vi "kill broken bundle.vi"(8 "error in":errorcluster, 11 "VI in":refnum<vi>) -> (0 "error out":errorcluster)   [LabVIEW 2013, in "FixedChannelTBModuleDecideFeatures.lvclass"]
uses:
  FixedChannelTBModuleDecideFeatures.lvclass
  <vilib>/Utility/traverseref.llb/TRef TravTarget.ctl
  <vilib>/Utility/traverseref.llb/VI Scripting - Traverse.lvlib
  <vilib>/Utility/VariantDataType/VariantType.lvlib
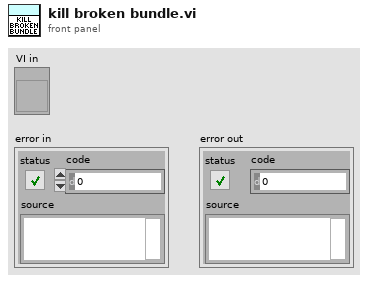
[diagram p1: front panel]
types:
  T1 = typedef "TRef TravTarget.ctl" = enum16{"FP", "BD", "Other"}
  T2 = typedef "VariantType.lvlib/Type.ctl" = enum8{"Invalid Type", "Void", "I8", "I16", "I32", "I64", "U8", "U16", "U32", "U64", "Single Float", "Double Float", "Extended Float", "Single Complex", "Double Complex", "Extended Complex", "Enum U8", "Enum U16", "Enum U32", "Enum U64", "Single Float With Unit", "Double Float With Unit", "Extended Float With Unit", "Single Complex with Unit", "Double Complex with Unit", "Extended Complex with Unit", "Boolean", "String", "Path", "Picture", "Tag", "Array", "Cluster", "Variant", "LV Variant", "Waveform", "Timestamp", "Digital Waveform", "Digital Data", "ExpressData", "Refnum", "External Data", "VI", "Poly VI", "LabVIEW Class Instance", "Fixed Point"}
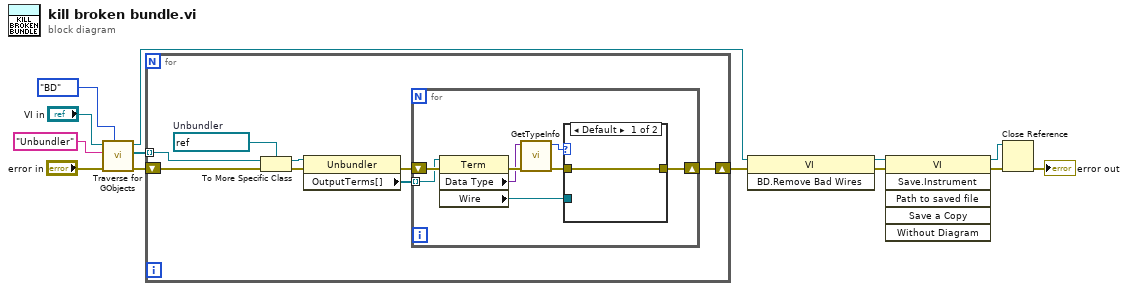
[diagram p0: block diagram]
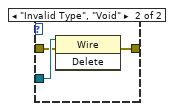
[diagram p2: hidden frame]
diagram:
  n1 = call <vilib>:"Traverse for GObjects.vi"("Traverse Target"=TRef_TravTarget."BD", "error in (no error)"="error in", "Class Name"="Unbundler", "VI Refnum"="VI in") -> ("error out"=w7:errorcluster, "References"=w6:refnum<vi>[], "dup VI Refnum"=w3:refnum<vi>)  [unwired: 4 in, 1 out]
  n2 = for {
    shift-right: [w15] -> w5
    shift-left: w7 -> [w20]
    tunnel: w6 -> [w19] mode=indexing
    w21 = refnum<vi> refnum  # Unbundler
    n3 = To More Specific Class(target class=w21, reference=w19, error in=w20) -> (specific class reference=w18:refnum<vi>, error out=w17:errorcluster)
    n4 = property class="Unbundler"(reference=w18, error in=w17) -> (error out=w16:errorcluster, "OutputTerms[]"=w14:refnum<vi>[])  [unwired: 1 out]
    n5 = for {
      shift-right: [w28] -> w15
      shift-left: w16 -> [w29]
      tunnel: w14 -> [w22] mode=indexing
      n6 = property class="Term"(reference=w22, error in=w29) -> (error out=w27:errorcluster, "Data Type"=w23:variant, "Wire"=w26:refnum<vi>)  [unwired: 1 out]
      n7 = call <vilib>:"GetTypeInfo.vi"("error in (no error)"=w27, "Variant"=w23) -> ("error out"=w25:errorcluster, "Type Enum"=w24:T2)  [unwired: 5 in, 3 out]
      n8 = case shown="Default" w24 {
        tunnel: [w30 w33] -> w28
        tunnel: w26 -> [_ w32]
        tunnel: w25 -> [w30 w31]
        frame Default {
        }
        frame "Invalid Type", "Void" {
          n9 = invoke class="Wire" method="Delete"(reference=w32, error in=w31) -> (error out=w33:errorcluster)  [unwired: 1 in, 2 out]
        }
      }
    }
  }
  n10 = invoke class="VI" method="BD.Remove Bad Wires"(reference=w3, error in=w5) -> (reference out=w2:refnum<vi>, error out=w4:errorcluster)  [unwired: 1 in, 1 out]
  n11 = invoke class="VI" method="Save.Instrument"(reference=w2, error in=w4) -> (reference out=w9:refnum<vi>, error out=w10:errorcluster)  [unwired: 4 in, 4 out]
  n12 = Close Reference(reference=w9, error in (no error)=w10) -> (error out=→"error out":errorcluster)
